vi "Main.vi"(8 "error in (no error)":errorcluster, 11 "ModuleAdmin":refnum<class "ModuleAdmin.lvclass">) -> ()   [LabVIEW 2014, in "AnalysisModule.lvlib"]
uses:
  AnalysisModule.lvlib
  <userlib>/NIST/ModuleAdminLib/ModuleAdmin/ModuleAdmin.lvclass
  AnalysisPlugins/AnalysisPluginBaseClass/Typedefs/clSensorData.ctl
  AnalysisPlugins/AnalysisPluginBaseClass/AnalysisPluginsBase.lvclass/AnalysisPluginsBase.ctl
  PublicAPI/Arguments/Requests/clStopArgument.ctl
  AnalysisPlugins/AnalysisPluginBaseClass/Typedefs/clSampleData.ctl
  AnalysisPlugins/AnalysisPluginBaseClass/Typedefs/clAnalysisConfig.ctl
  AnalysisPlugins/AnalysisPluginBaseClass/Typedefs/SignalParams.ctl
  <userlib>/NIST/ModuleAdminLib/ModuleAdmin/ModuleAdmin.lvclass/ModuleAdmin.ctl
  AnalysisPlugins/AnalysisPluginBaseClass/AnalysisPluginsBase.lvclass
  <userlib>/NIST/BaseClasses/BasePlugin_class/BasePlugin.lvclass/BasePlugin.ctl
  <vilib>/Utility/error.llb/DialogType.ctl
  AnalysisPlugins/AnalysisPluginBaseClass/Accessors/Read ResultArray.vi
  AnalysisPlugins/AnalysisPluginBaseClass/Accessors/Read SampleDataQueName.vi
  AnalysisPlugins/AnalysisPluginBaseClass/Accessors/Write clConfig.vi
  AnalysisPlugins/AnalysisPluginBaseClass/Accessors/Write MagCorr.vi
  AnalysisPlugins/AnalysisPluginBaseClass/Accessors/Write DelayCorr.vi
  AnalysisPlugins/AnalysisPluginBaseClass/Accessors/Write SignalParams.vi
  AnalysisPlugins/AnalysisPluginBaseClass/Accessors/Write TestType.vi
  AnalysisPlugins/AnalysisPluginBaseClass/Accessors/Write FileName.vi
  <userlib>/NIST/ModuleAdminLib/ModuleAdmin/Accessors/Read ShowPanel_.vi
  <userlib>/NIST/ModuleAdminLib/ModuleAdmin/Accessors/Write ShowPanel_.vi
  <userlib>/NIST/BaseClasses/BasePlugin_class/Accessors/Write PluginIniFilePath.vi
  AnalysisPlugins/AnalysisPluginBaseClass/Accessors/Write SampleDataQueName.vi
  <userlib>/NIST/BaseClasses/BasePlugin_class/Accessors/Read PluginIniFilePath.vi
  <userlib>/NIST/ModuleAdminLib/ModuleAdmin/Accessors/Read CloneRegRef.vi
  <vilib>/Utility/error.llb/Error Cluster From Error Code.vi
  <vilib>/ErrorRing/Error Ring.xnode
  <userlib>/NIST/ModuleAdminLib/CloneRegistration/CloneRegistration.lvclass
  <userlib>/NIST/ModuleAdminLib/ModuleAdmin.lvlib
  Sensor/SensorModule/SensorModule.lvlib
panel:
  out "error out":errorcluster
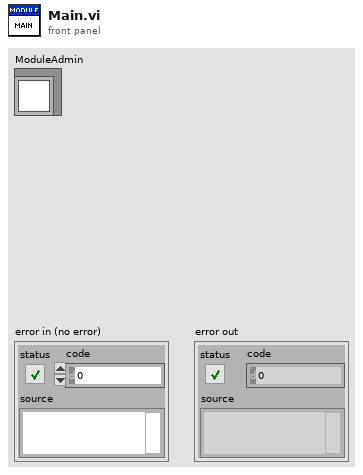
[diagram p1: front panel]
types:
  T1 = typedef "AnalysisPlugins.lvlib/AnalysisPluginsBase.lvclass/clSensorData.ctl" = cluster{"SensorType":string, "SensorData":variant}
  T2 = typedef "AnalysisModule.lvlib/clRequestEvents.ctl" = cluster{"StopRequest":refnum<user-event>, "PathToINI":refnum<user-event>, " LoadPlugin":refnum<user-event>, "ShowPanel":refnum<user-event>, "WriteSamples":refnum<user-event>, "ReadConfig":refnum<user-event>, "WriteConfig":refnum<user-event>, "WriteSignalParams":refnum<user-event>, "WriteTestType":refnum<user-event>, "WriteFileName":refnum<user-event>, "WriteMagCorr":refnum<user-event>, "WriteDlyCorr":refnum<user-event>}
  T3 = typedef "AnalysisModule.lvlib/clBroadcastEvents.ctl" = cluster{"DidInit":refnum<user-event>, "StatusUpdate":refnum<user-event>, "ErrorReport":refnum<user-event>, "DidStop":refnum<user-event>, "PathToINI":refnum<user-event>, "Config":refnum<user-event>, "ResultReport":refnum<user-event>}
  T4 = typedef "SensorModule.lvlib/clBroadcastEvents.ctl" = cluster{"DidInit":refnum<user-event>, "StatusUpdate":refnum<user-event>, "ErrorReport":refnum<user-event>, "DidStop":refnum<user-event>, "PathToINI":refnum<user-event>, "SensorReport":refnum<user-event>, "SensorConfig":refnum<user-event>}
  T5 = typedef "AnalysisModule.lvlib/clStopArgument.ctl" = cluster{"Exit via Stop Module Req?":bool, "Wait for Module to stop?":bool, "ModuleAdmin":refnum<class "ModuleAdmin.lvclass">}
  T6 = typedef "AnalysisPlugins.lvlib/AnalysisPluginsBase.lvclass/clAnalysisConfig.ctl" = cluster{"F0":u32, "SettlingTime":dbl, "AnalysisCycles":dbl, "SampleRate":dbl, "NumChannels":u32, "TsOffset":enum16{"start", "middle", "end"}}
  T7 = typedef "AnalysisPlugins.lvlib/AnalysisPluginsBase.lvclass/SignalParams.ctl" = dbl[]
  T8 = enum32{"Invalid", "Standard", "Closed", "Hidden", "Minimized", "Maximized"}
  T9 = typedef "AnalysisPlugins.lvlib/AnalysisPluginsBase.lvclass/clSampleData.ctl" = cluster{"Timestamp":ext, "SampleDataInput":cluster{"dSampleData":dbl[], "iActualPts":i32}[]}
  T10 = typedef "DialogType.ctl" = u16
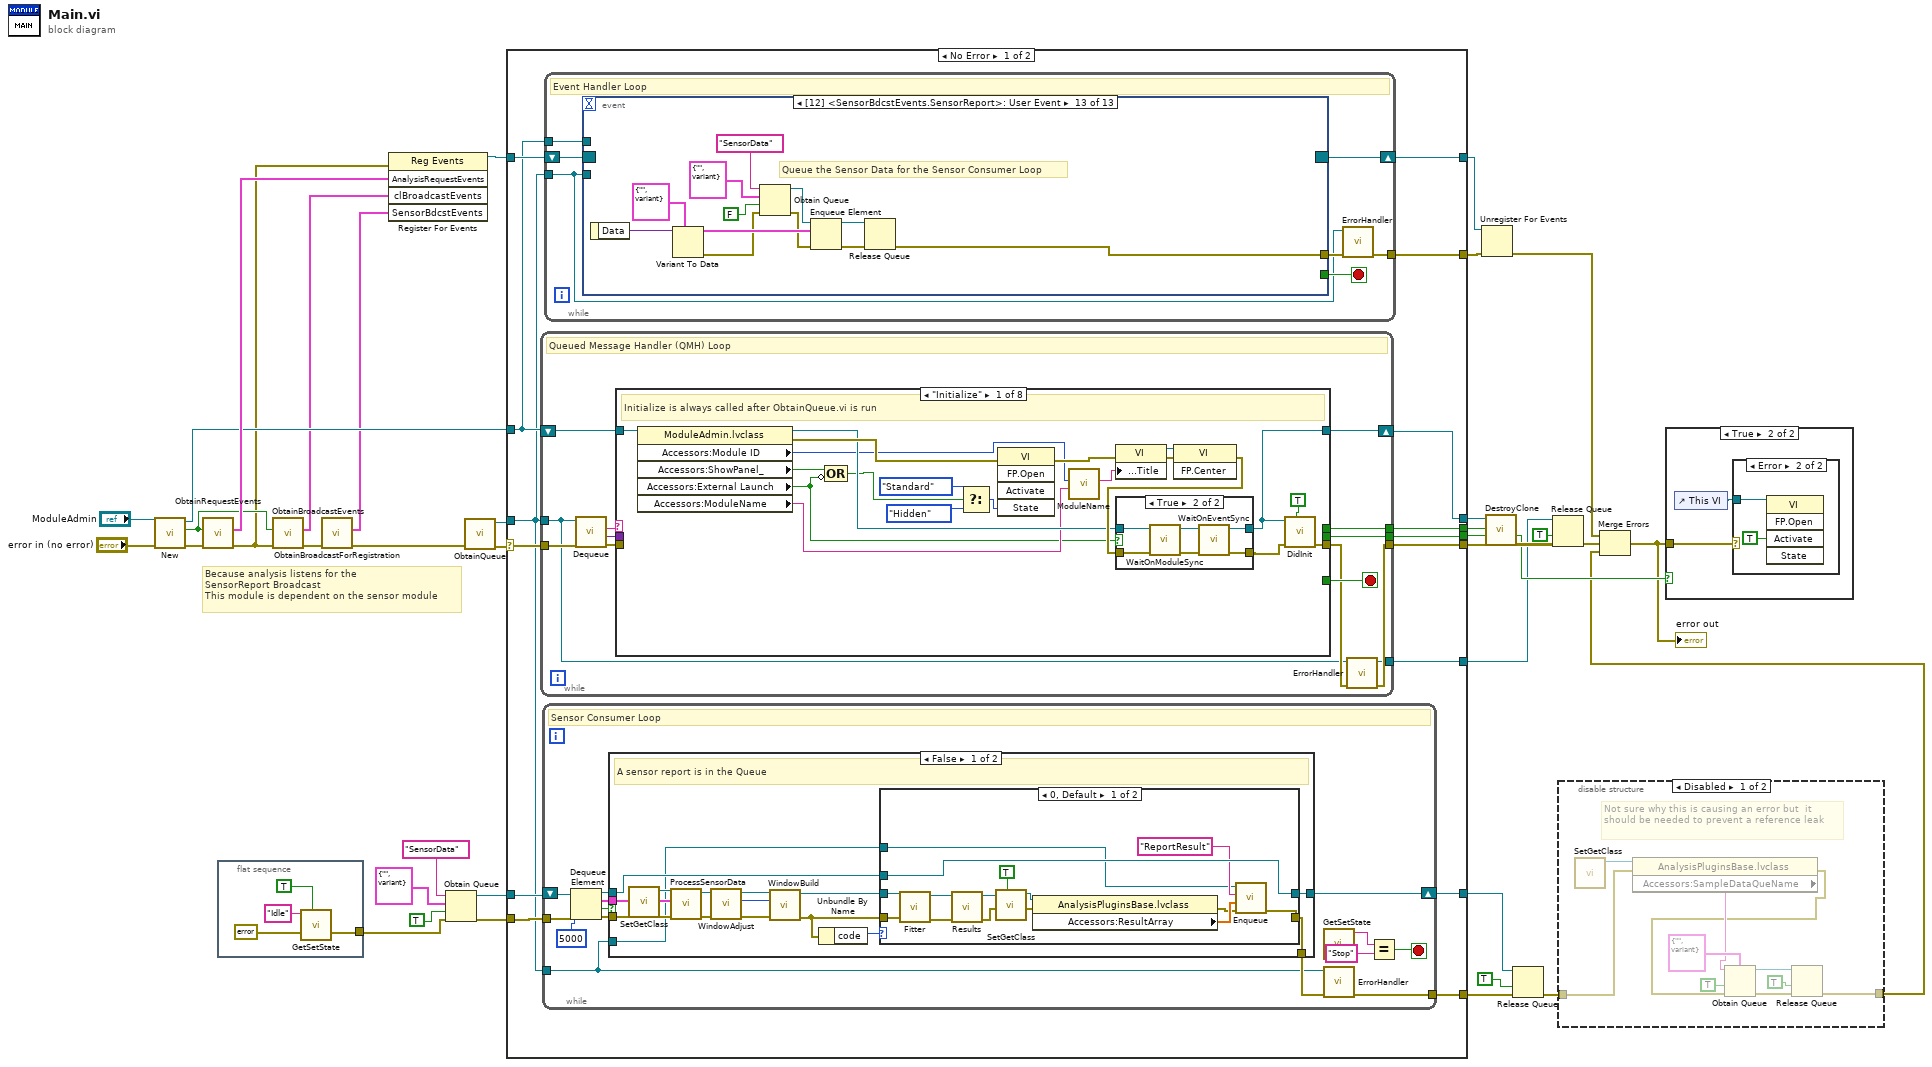
[diagram p0: block diagram]
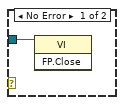
[diagram p4: hidden frame]
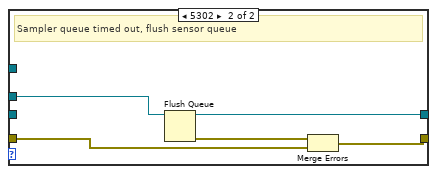
[diagram p5: hidden frame]
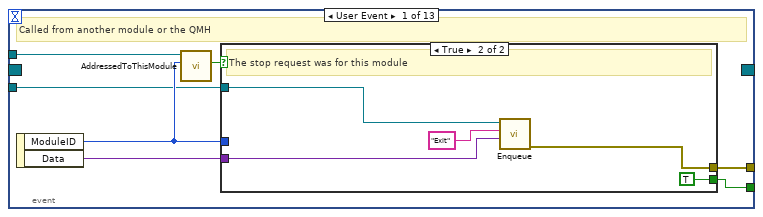
[diagram p7: hidden frame]
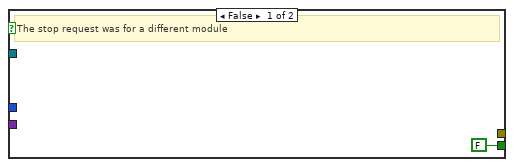
[diagram p8: hidden frame]
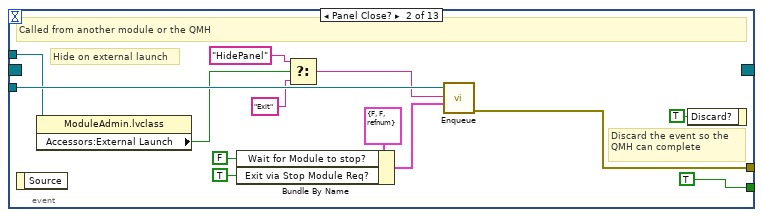
[diagram p9: hidden frame]
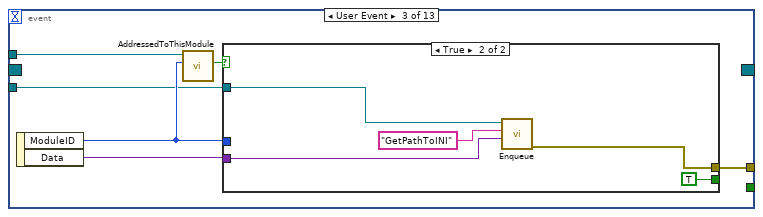
[diagram p10: hidden frame]
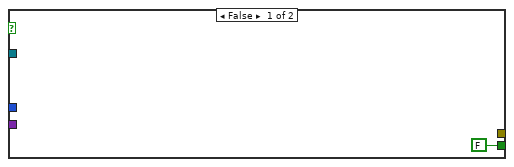
[diagram p11: hidden frame]
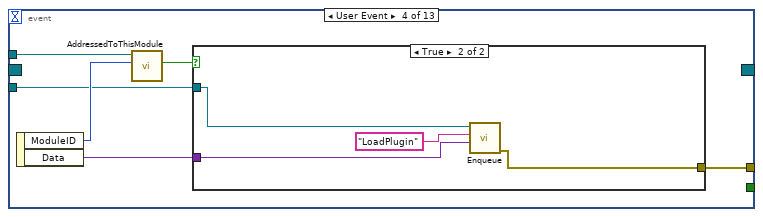
[diagram p12: hidden frame]
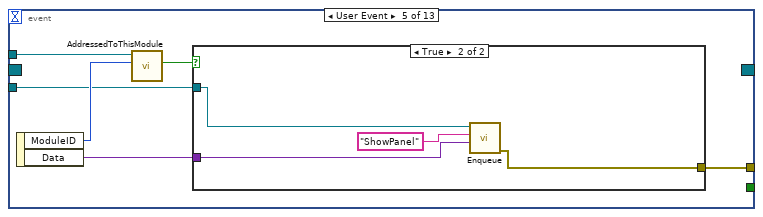
[diagram p14: hidden frame]
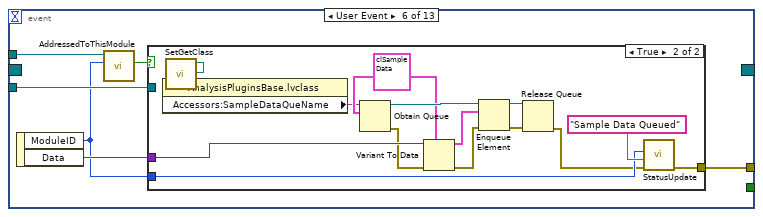
[diagram p16: hidden frame]
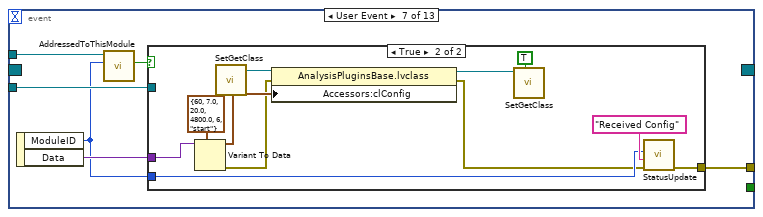
[diagram p18: hidden frame]
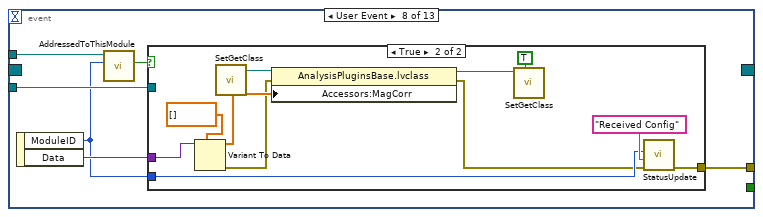
[diagram p20: hidden frame]
diagram:
  # "Because analysis listens for the\nSensorReport Broadcast\nThis module is dependent on the sensor module"
  n1 = call <userlib>:"New.vi"("error in (no error)"="error in (no error)", "ModuleAdmin"="ModuleAdmin") -> ("error out"=w36:errorcluster, "First?"=w31:bool, "ModuleAdmin"=w32:refnum<class "ModuleAdmin.lvclass">)  [unwired: 7 in]
  n2 = call "ObtainRequestEvents.vi"("error in (no error)"=w36, "CreateNew (F)"=w31) -> ("error out"=w30:errorcluster, "AnalysisRequestEvents"=w35:T2)  [unwired: 8 in]
  n3 = flat-sequence {
    tunnel: [errorcluster {"status"=FALSE, "code"=0, "source"=""} ("error constant")] -> w15
    frame #0 {
      n4 = call "GetSetState.vi"("Set (f)"=TRUE, "State In"="Idle") -> ()  [unwired: 9 in, 1 out]
    }
  }
  n5 = call "ObtainBroadcastEvents.vi"("error in (no error)"=w30, "CreateNew? (F)"=w31) -> ("error out"=w14:errorcluster, "clBroadcastEvents"=w29:T3)  [unwired: 8 in]
  n6 = call "ObtainBroadcastForRegistration.vi"("error in (no error)"=w14) -> ("error out"=w13:errorcluster, "SensorBdcstEvents"=w12:T4)  [unwired: 9 in]
  n7 = register-events(error in=w30, w35, w29, w12) -> (reference out=w28:refnum<event-registration>)  [unwired: 1 in, 1 out]
  n8 = Obtain Queue(name (unnamed)="SensorData", element data type=T1 {"SensorType"="", "SensorData"=variant} ("clSensorData"), create if not found? (T)=TRUE, error in (no error)=w15) -> (queue out=w17:refnum<queue>, error out=w16:errorcluster)  [unwired: 1 in, 1 out]
  n9 = call "ObtainQueue.vi"("error in (no error)"=w13) -> ("error out"=w34:errorcluster, "MessageQueue"=w33:refnum<queue>)  [unwired: 9 in]
  n10 = case shown="No Error" w34 {
    selector: w34 -> [w56 w477]
    tunnel: w33 -> [w46 w467]
    tunnel: w32 -> [w53 w474]
    tunnel: [w55 w475] -> w27
    tunnel: w28 -> [w54 w469]
    tunnel: [w52 w473] -> w25
    tunnel: [w51 _] -> w24
    tunnel: [w50 _] -> w23
    tunnel: [w49 _] -> w11
    tunnel: w17 -> [w48 w468]
    tunnel: w16 -> [w47 w470]
    tunnel: [w45 w470] -> w6
    tunnel: [w44 w469] -> w10
    tunnel: [w43 w468] -> w3
    tunnel: [w42 w467] -> w2
    frame No Error {
      n11 = while {
        tunnel: w46 -> [w310]
        tunnel: w56 -> [w319]
        tunnel: [w312] -> w55
        tunnel: [w314] -> w51
        tunnel: [w313] -> w50
        shift-right: [w309] -> w52
        shift-left: w53 -> [w315]
        tunnel: [w308] -> w42
        stop <- w320 stop-if-true
        # "Queued Message Handler (QMH) Loop"
        n12 = call "Dequeue.vi"("error in (no error)"=w319, "MessageQueue"=w310) -> ("error out"=w318:errorcluster, "Message Data"=w316:variant, "Message"=w317:string)  [unwired: 6 in, 1 out]
        n13 = case shown="\"Initialize\"" w317 {
          selector: w317 -> [_ _ _ _ _ _ _ w455]
          tunnel: [_ _ _ _ _ w427 _ _] -> w320
          tunnel: w315 -> [w340 w356 w368 w416 w426 w429 w437 w458]
          tunnel: [w330 w349 w369 w417 w419 w435 w438 w454] -> w311
          tunnel: w318 -> [_ w359 w373 w414 w425 w434 w446 _]
          tunnel: w316 -> [_ w358 w375 _ _ w433 w445 _]
          tunnel: [_ _ _ _ _ w431 _ _] -> w314
          tunnel: [_ _ _ _ _ w430 _ _] -> w313
          tunnel: [w323 w355 w367 w412 w424 w429 w436 w452] -> w309
          frame "Initialize" {
            # "Initialize is always called after ObtainQueue.vi is run"
            n14 = property class="ModuleAdmin.lvclass"(reference=w340) -> (reference out=w328:refnum<class "ModuleAdmin.lvclass">, error out=w337:errorcluster, "Accessors:Module ID"=w322:i32, "Accessors:ShowPanel_"=w326:bool, "Accessors:External Launch"=w325:bool, "Accessors:ModuleName"=w327:string)  [unwired: 1 in]
            n15 = Compound Arithmetic op=OR(w326, invert w325) -> (w324:bool)
            n16 = Select(t=T8."Standard" ("Front Panel Window:State"), s=w324, f=T8."Hidden" ("Front Panel Window:State")) -> (s? t:f=w333:T8)
            n17 = invoke class="VI" method="FP.Open"(error in=w337, "State"=w333) -> (error out=w336:errorcluster)  [unwired: 3 in, 4 out]
            n18 = call <userlib>:"ModuleName.vi"("Name"=w327, "ModuleID"=w322) -> ("ModuleName"=w332:string)  [unwired: 9 in]
            n19 = property class="VI"(error in=w336, "Front Panel.Title"=w332) -> (reference out=w339:refnum<vi>, error out=w338:errorcluster)  [unwired: 1 in]
            n20 = invoke class="VI" method="FP.Center"(reference=w339, error in=w338) -> (error out=w329:errorcluster)  [unwired: 1 in, 2 out]
            n21 = case shown="True" w325 {
              tunnel: [w341 w347] -> w321
              tunnel: [w342 w344] -> w323
              tunnel: w329 -> [w341 w346]
              tunnel: w328 -> [w342 w343]
              frame False {
              }
              frame True {
                n22 = call <userlib>:"WaitOnModuleSync.vi"("error in (no error)"=w346, "ModuleAdmin"=w343) -> ("error out"=w348:errorcluster, "ModuleAdmin"=w345:refnum<class "ModuleAdmin.lvclass">)  [unwired: 8 in]
                n23 = call <userlib>:"WaitOnEventSync.vi"("error in (no error)"=w348, "ModuleAdmin"=w345) -> ("error out"=w347:errorcluster, "ModuleAdmin"=w344:refnum<class "ModuleAdmin.lvclass">)  [unwired: 8 in]
              }
            }
            n24 = call "DidInit.vi"("Init?"=TRUE, "error in (no error)"=w321, "ModuleAdmin"=w323) -> ("error out"=w330:errorcluster)  [unwired: 8 in]
          }
          frame "ShowPanel" {
            n25 = Variant To Data(error in=w359, type=TRUE, Variant=w358) -> (data=w351:bool, error out=w354:errorcluster)
            n26 = Select(t=T8."Standard" ("Front Panel Window:State"), s=w351, f=T8."Hidden" ("Front Panel Window:State")) -> (s? t:f=w350:T8)
            n27 = property class="VI"(error in=w354, "FP.State"=w350) -> (error out=w349:errorcluster)  [unwired: 1 in, 1 out]
            n28 = property class="ModuleAdmin.lvclass"(reference=w356, "Accessors:ShowPanel_"=w351) -> (reference out=w355:refnum<class "ModuleAdmin.lvclass">)  [unwired: 1 in, 1 out]
          }
          frame "LoadPlugin" {
            n29 = Variant To Data(error in=w373, type=path "", Variant=w375) -> (data=w364:path, error out=w363:errorcluster)
            n30 = call "GetDefaultParams.vi"("error in (no error)"=w363, "PathToIni"=w364) -> ("error out"=w362:errorcluster, "clConfig"=w360:T6, "PathToClass"=w361:path)  [unwired: 7 in]
            n31 = call <vilib>:"Check if File or Folder Exists.vi"("error in (no error)"=w362, "path"=w361) -> ("error out"=w370:errorcluster, "file or folder exists?"=w372:bool, "dup path"=w371:path)  [unwired: 7 in]
            n32 = case shown="True" w372 {
              tunnel: w371 -> [w381 w403]
              tunnel: w370 -> [w376 w410]
              tunnel: [w377 w406] -> w369
              tunnel: w368 -> [w380 w405]
              tunnel: [refnum<class "AnalysisPluginsBase.lvclass"> refnum ("AnalysisPlugins.lvlib:AnalysisPluginsBase.lvclass") w391] -> w366
              tunnel: w364 -> [_ w401]
              tunnel: [w380 w400] -> w367
              tunnel: w360 -> [_ w392]
              frame False {
                n33 = Path To String(path=w381) -> (string=w382:string)
                n34 = xnode "Error Ring"("parameter 0"=w382) -> ("error out"=w378:errorcluster)
                n35 = Merge Errors(w376, w378) -> (w377:errorcluster)
              }
              frame True {
                n36 = call-dynamic "LoadClassFromFile.vi"("error in (no error)"=w410, "class path"=w403, "reference in"=refnum<class "AnalysisPluginsBase.lvclass"> refnum) -> ("error out"=w402:errorcluster, "reference out"=w404:refnum<class "AnalysisPluginsBase.lvclass">)  [unwired: 7 in]
                n37 = property class="ModuleAdmin.lvclass"(reference=w405) -> (reference out=w400:refnum<class "ModuleAdmin.lvclass">, "Accessors:Module ID"=w396:i32)  [unwired: 1 in, 1 out]
                n38 = Number To Decimal String(number=w396) -> (decimal integer string=w398:string)  [unwired: 1 in]
                n39 = Concatenate Strings("SampleData" ("name (unnamed)"), w398) -> (w393:string)
                n40 = Obtain Queue(name (unnamed)=w393, element data type=T9 {"Timestamp"=0.0, "SampleDataInput"=[]} ("clSampleData"), create if not found? (T)=TRUE) -> ()  [unwired: 2 in, 3 out]
                n41 = property class="AnalysisPluginsBase.lvclass"(reference=w404, error in=w402, "Accessors:PluginIniFilePath"=w401, "Accessors:SampleDataQueName"=w393, "Accessors:clConfig"=w392) -> (reference out=w391:refnum<class "AnalysisPluginsBase.lvclass">, error out=w390:errorcluster)
                n42 = Path To String(path=w403) -> (string=w408:string)
                n43 = Format Into String(format string="Plugin %s loaded ", w408) -> (resulting string=w407:string)  [unwired: 2 in, 1 out]
                n44 = call "StatusUpdate.vi"("error in (no error)"=w390, "Status"=w407, "ModuleID"=w396) -> ("error out"=w406:errorcluster)  [unwired: 8 in]
              }
            }
            n45 = call "SetGetClass.vi"("Set (f)"=TRUE, "Analysis In"=w366) -> ()  [unwired: 9 in, 1 out]
          }
          frame "GetPathToINI" {
            n46 = call "SetGetClass.vi"() -> ("Analysis Out"=w411:refnum<class "AnalysisPluginsBase.lvclass">)  [unwired: 11 in]
            n47 = property class="AnalysisPluginsBase.lvclass"(reference=w411, error in=w414) -> (error out=w413:errorcluster, "Accessors:PluginIniFilePath"=w415:path)  [unwired: 1 out]
            n48 = property class="ModuleAdmin.lvclass"(reference=w416) -> (reference out=w412:refnum<class "ModuleAdmin.lvclass">, "Accessors:Module ID"=w418:i32)  [unwired: 1 in, 1 out]
            n49 = call "PathToINIBroadcast.vi"("error in (no error)"=w413, "PathToINI"=w415, "ModuleID"=w418) -> ("error out"=w417:errorcluster)  [unwired: 8 in]
          }
          frame "ReportResult" {
            n50 = call "SetGetClass.vi"() -> ("Analysis Out"=w423:refnum<class "AnalysisPluginsBase.lvclass">)  [unwired: 11 in]
            n51 = property class="AnalysisPluginsBase.lvclass"(reference=w423, error in=w425) -> (error out=w420:errorcluster, "Accessors:ResultArray"=w421:dbl[])  [unwired: 1 out]
            n52 = property class="ModuleAdmin.lvclass"(reference=w426) -> (reference out=w424:refnum<class "ModuleAdmin.lvclass">, "Accessors:Module ID"=w422:i32)  [unwired: 1 in, 1 out]
            n53 = call "ReportResults.vi"("error in (no error)"=w420, "ResultsArray"=w421, "ModuleID"=w422) -> ("error out"=w419:errorcluster)  [unwired: 8 in]
          }
          frame "Exit" {
            w427 = TRUE
            # "Called by the StopRequest event handler case"
            n54 = control-ref of="This VI"() -> (w432:refnum<vi>)
            n55 = call "HandleExit.vi"("error in (no error)"=w434, "VI Refnum"=w432, "StopArgument"=w433, "ModuleAdmin"=w429) -> ("error out"=w435:errorcluster, "Exit via Stop Module Req?"=w430:bool, "WaitForStop?"=w431:bool)  [unwired: 5 in]
            n56 = call "GetSetState.vi"("Set (f)"=w427, "State In"="Stop") -> ()  [unwired: 9 in, 1 out]
          }
          frame "Error" {
            n57 = property class="ModuleAdmin.lvclass"(reference=w437) -> (reference out=w436:refnum<class "ModuleAdmin.lvclass">, "Accessors:External Launch"=w441:bool, "Accessors:Module ID"=w439:i32)  [unwired: 1 in, 1 out]
            n58 = Variant To Data(error in=w446, type=errorcluster {"status"=FALSE, "code"=0, "source"=""} ("error constant"), Variant=w445) -> (data=w440:errorcluster, error out=w443:errorcluster)
            n59 = call "ReportError.vi"("error in (no error)"=w443, "ErrorReported"=w440, "ModuleID"=w439) -> ("error out"=w442:errorcluster)  [unwired: 8 in]
            n60 = case shown="False" w441 {
              tunnel: w442 -> [w450 w451]
              tunnel: w440 -> [w449 _]
              tunnel: [w448 w451] -> w438
              tunnel: w437 -> [w447 _]
              frame False {
                # "Todo:  Add an event to ask the user\nIf the module should stop or continue"
                # "Stand alone: now, force an exit"
                n61 = call <vilib>:"Simple Error Handler.vi"("error in (no error)"=w449) -> ()  [unwired: 4 in, 5 out]
                n62 = call "StopRequest.vi"("error in (no error)"=w450, "ModuleAdmin"=w447) -> ("error out"=w448:errorcluster)  [unwired: 8 in, 1 out]
              }
              frame True {
                # "Externally launched modules only broadcast the error msg"
              }
            }
          }
          frame Default {
            # "Called only if a message was queued and no QMH case was created"
            n63 = property class="ModuleAdmin.lvclass"(reference=w458) -> (reference out=w452:refnum<class "ModuleAdmin.lvclass">, "Accessors:Module ID"=w457:i32, "Accessors:ModuleName"=w453:string)  [unwired: 1 in, 1 out]
            n64 = call <userlib>:"ModuleName.vi"("Name"=w453, "ModuleID"=w457) -> ("ModuleName"=w456:string)  [unwired: 9 in]
            n65 = xnode "Error Ring"("parameter 0"=w455, "parameter 1"=w456) -> ("error out"=w454:errorcluster)
          }
        }
        n66 = call "ErrorHandler.vi"("error in (no error)"=w311, "MessageQueue"=w310) -> ("error out"=w312:errorcluster, "MessageQueue"=w308:refnum<queue>)  [unwired: 8 in]
      }
      n67 = while {
        tunnel: w47 -> [w63]
        tunnel: w46 -> [w57]
        tunnel: [w61] -> w45
        shift-right: [w58] -> w43
        shift-left: w48 -> [w60]
        stop <- w68 stop-if-true
        # "Sensor Consumer Loop"
        n68 = Dequeue Element(queue=w60, timeout in ms (-1)=5000, error in (no error)=w63) -> (queue out=w59:refnum<queue>, element=w65:T1, timed out?=w66:bool, error out=w64:errorcluster)
        n69 = case shown="False" w66 {
          tunnel: w65 -> [w77 _]
          tunnel: w64 -> [w85 w106]
          tunnel: [w74 w106] -> w62
          tunnel: w59 -> [w73 w105]
          tunnel: [w72 w105] -> w58
          tunnel: w57 -> [w71 _]
          frame False {
            # "A sensor report is in the Queue"
            n70 = call "SetGetClass.vi"() -> ("Analysis Out"=w84:refnum<class "AnalysisPluginsBase.lvclass">)  [unwired: 11 in]
            n71 = call-dynamic "ProcessSensorData.vi"("error in (no error)"=w85, "clSensorData"=w77, "Class In"=w84) -> ("error out"=w83:errorcluster, "Class Out"=w82:refnum<class "AnalysisPluginsBase.lvclass">)  [unwired: 7 in]
            n72 = call "WindowAdjust.vi"("error in (no error)"=w83, "AnalysisPluginsBase in"=w82) -> ("error out"=w81:errorcluster, "SamplesNeeded"=w79:u32, "AnalysisPluginsBase out"=w80:refnum<class "AnalysisPluginsBase.lvclass">)  [unwired: 7 in]
            n73 = call "WindowBuild.vi"("error in (no error)"=w81, "SamplesNeeded"=w79, "AnalysisPluginsBase in"=w80) -> ("error out"=w75:errorcluster, "AnalysisPluginsBase out"=w76:refnum<class "AnalysisPluginsBase.lvclass">)  [unwired: 7 in]
            n74 = Unbundle By Name(w75) -> ("code"=w78:i32)
            n75 = case shown="0, Default" w78 {
              tunnel: w76 -> [w96 _]
              tunnel: w75 -> [w97 w100]
              tunnel: [w92 w104] -> w74
              tunnel: w73 -> [w98 w103]
              tunnel: [w98 w101] -> w72
              tunnel: w71 -> [w86 _]
              frame 0, Default {
                n76 = call-dynamic "Fitter.vi"("error in (no error)"=w97, "AnalysisPluginsBase in"=w96) -> ("error out"=w95:errorcluster, "AnalysisPluginsBase out"=w94:refnum<class "AnalysisPluginsBase.lvclass">)  [unwired: 8 in]
                n77 = call-dynamic "Results.vi"("error in (no error)"=w95, "AnalysisPluginsBase in"=w94) -> ("error out"=w88:errorcluster, "AnalysisPluginsBase out"=w93:refnum<class "AnalysisPluginsBase.lvclass">)  [unwired: 8 in]
                n78 = call "SetGetClass.vi"("Set (f)"=TRUE, "Analysis In"=w93) -> ("Analysis Out"=w91:refnum<class "AnalysisPluginsBase.lvclass">)  [unwired: 9 in]
                n79 = property class="AnalysisPluginsBase.lvclass"(reference=w91, error in=w88) -> (error out=w87:errorcluster, "Accessors:ResultArray"=w90:dbl[])  [unwired: 1 out]
                n80 = call "Enqueue.vi"("error in (no error)"=w87, "Message Data"=w90, "Message"="ReportResult", "MessageQueue"=w86) -> ("error out"=w92:errorcluster)  [unwired: 6 in, 1 out]
              }
              frame 5302 {
                # "Sampler queue timed out, flush sensor queue"
                n81 = Flush Queue(queue=w103) -> (queue out=w101:refnum<queue>, error out=w102:errorcluster)  [unwired: 1 in, 1 out]
                n82 = Merge Errors(w102, w100) -> (w104:errorcluster)
              }
            }
          }
          frame True {
            # "Queue Timed out, allow the loop to run to check for Stop State"
          }
        }
        n83 = call "GetSetState.vi"() -> ("State Out"=w70:string)  [unwired: 11 in]
        n84 = call "ErrorHandler.vi"("error in (no error)"=w62, "MessageQueue"=w57) -> ("error out"=w61:errorcluster)  [unwired: 8 in, 1 out]
        n85 = Equal?(x=w70, y="Stop") -> (x = y?=w68:bool)
      }
      n86 = while {
        tunnel: w46 -> [w107]
        shift-right: [w111] -> w44
        shift-left: w54 -> [w112]
        tunnel: w53 -> [w110]
        tunnel: [w108] -> w49
        stop <- w113 stop-if-true
        # "Event Handler Loop"
        n87 = event shown="[12] <SensorBdcstEvents.SensorReport>: User Event" {
          selector: w112 -> [_ _ _ _ _ _ _ _ _ _ _ _ _]
          dyn-events: [_ _ _ _ _ _ _ _ _ _ _ _ _] -> w111
          timeout: _ -> [_ _ _ _ _ _ _ _ _ _ _ _ _]
          tunnel: w107 -> [w117 w139 w142 w153 w163 w175 w195 w212 w229 w246 w263 w280 _]
          tunnel: [w116 TRUE _ _ _ _ _ _ _ _ _ _ _] -> w113
          tunnel: w110 -> [w120 w133 w141 w157 w167 w177 w197 w214 w231 w248 w265 w282 _]
          tunnel: [w115 w137 w140 w154 w164 w173 w193 w210 w227 w244 w261 w278 w297] -> w109
          event User Event {
            # "Called from another module or the QMH"
            n88 = event-data() -> ("ModuleID"=w118:i32, "Data"=w114:variant)  [unwired: 1 in]
            n89 = call <userlib>:"AddressedToThisModule.vi"("ModuleID"=w118, "ModuleAdmin"=w120) -> ("AddressedToThisInstance?"=w119:bool)  [unwired: 8 in, 1 out]
            n90 = case shown="True" w119 {
              tunnel: w118 -> [_ _]
              tunnel: w117 -> [_ w126]
              tunnel: [FALSE TRUE] -> w116
              tunnel: [_ w124] -> w115
              tunnel: w114 -> [_ w122]
              frame False {
                # "The stop request was for a different module"
              }
              frame True {
                # "The stop request was for this module"
                n91 = call "Enqueue.vi"("Message Data"=w122, "Message"="Exit", "MessageQueue"=w126) -> ("error out"=w124:errorcluster)  [unwired: 7 in, 1 out]
              }
            }
          }
          event Panel Close? {
            # "Hide on external launch"
            # "Discard the event so the QMH can complete"
            # "Called from another module or the QMH"
            n92 = event-data() -> ()  [unwired: 1 in, 1 out]
            n93 = property class="ModuleAdmin.lvclass"(reference=w133) -> ("Accessors:External Launch"=w128:bool)  [unwired: 1 in, 2 out]
            n94 = Bundle By Name(cluster=T5 {"Exit via Stop Module Req?"=FALSE, "Wait for Module to stop?"=FALSE, "ModuleAdmin"=refnum} ("Stop Argument"), "Wait for Module to stop?"=FALSE, "Exit via Stop Module Req?"=TRUE) -> (w134:T5)
            n95 = Select(t="HidePanel", s=w128, f="Exit" ("Message")) -> (s? t:f=w130:string)
            n96 = call "Enqueue.vi"("Message Data"=w134, "Message"=w130, "MessageQueue"=w139) -> ("error out"=w137:errorcluster)  [unwired: 7 in, 1 out]
            n97 = event-data("Discard?"=TRUE) -> ()  [unwired: 1 in, 1 out]
          }
          event User Event {
            n98 = event-data() -> ("ModuleID"=w143:i32, "Data"=w144:variant)  [unwired: 1 in]
            n99 = call <userlib>:"AddressedToThisModule.vi"("ModuleID"=w143, "ModuleAdmin"=w141) -> ("AddressedToThisInstance?"=w145:bool)  [unwired: 8 in, 1 out]
            n100 = case shown="True" w145 {
              tunnel: w143 -> [_ _]
              tunnel: w142 -> [_ w151]
              tunnel: [FALSE TRUE] -> _
              tunnel: [_ w149] -> w140
              tunnel: w144 -> [_ w147]
              frame False {
                # "The stop request was for a different module"
              }
              frame True {
                # "The stop request was for this module"
                n101 = call "Enqueue.vi"("Message Data"=w147, "Message"="GetPathToINI", "MessageQueue"=w151) -> ("error out"=w149:errorcluster)  [unwired: 7 in, 1 out]
              }
            }
          }
          event User Event {
            n102 = event-data() -> ("ModuleID"=w156:i32, "Data"=w152:variant)  [unwired: 1 in]
            n103 = call <userlib>:"AddressedToThisModule.vi"("ModuleID"=w156, "ModuleAdmin"=w157) -> ("AddressedToThisInstance?"=w155:bool)  [unwired: 8 in, 1 out]
            n104 = case shown="True" w155 {
              tunnel: [_ w158] -> w154
              tunnel: w153 -> [_ w161]
              tunnel: w152 -> [_ w159]
              frame False {
              }
              frame True {
                n105 = call "Enqueue.vi"("Message Data"=w159, "Message"="LoadPlugin", "MessageQueue"=w161) -> ("error out"=w158:errorcluster)  [unwired: 7 in, 1 out]
              }
            }
          }
          event User Event {
            n106 = event-data() -> ("ModuleID"=w166:i32, "Data"=w162:variant)  [unwired: 1 in]
            n107 = call <userlib>:"AddressedToThisModule.vi"("ModuleID"=w166, "ModuleAdmin"=w167) -> ("AddressedToThisInstance?"=w165:bool)  [unwired: 8 in, 1 out]
            n108 = case shown="True" w165 {
              tunnel: [_ w168] -> w164
              tunnel: w163 -> [_ w171]
              tunnel: w162 -> [_ w169]
              frame False {
              }
              frame True {
                n109 = call "Enqueue.vi"("Message Data"=w169, "Message"="ShowPanel", "MessageQueue"=w171) -> ("error out"=w168:errorcluster)  [unwired: 7 in, 1 out]
              }
            }
          }
          event User Event {
            n110 = event-data() -> ("ModuleID"=w172:i32, "Data"=w174:variant)  [unwired: 1 in]
            n111 = call <userlib>:"AddressedToThisModule.vi"("ModuleID"=w172, "ModuleAdmin"=w177) -> ("AddressedToThisInstance?"=w176:bool)  [unwired: 8 in, 1 out]
            n112 = case shown="True" w176 {
              tunnel: w175 -> [_ _]
              tunnel: w174 -> [_ w191]
              tunnel: [_ w184] -> w173
              tunnel: w172 -> [_ w183]
              frame False {
              }
              frame True {
                w188 = T9 {"Timestamp"=0.0, "SampleDataInput"=[]} ("clSampleData")
                n113 = call "SetGetClass.vi"() -> ("Analysis Out"=w182:refnum<class "AnalysisPluginsBase.lvclass">)  [unwired: 11 in]
                n114 = property class="AnalysisPluginsBase.lvclass"(reference=w182) -> ("Accessors:SampleDataQueName"=w181:string)  [unwired: 1 in, 2 out]
                n115 = Obtain Queue(name (unnamed)=w181, element data type=w188) -> (queue out=w189:refnum<queue>, error out=w187:errorcluster)  [unwired: 3 in, 1 out]
                n116 = Variant To Data(error in=w187, type=w188, Variant=w191) -> (data=w190:T9, error out=w186:errorcluster)
                n117 = Enqueue Element(queue=w189, element=w190, error in (no error)=w186) -> (queue out=w178:refnum<queue>, error out=w180:errorcluster)  [unwired: 1 in, 1 out]
                n118 = Release Queue(queue=w178, error in (no error)=w180) -> (error out=w179:errorcluster)  [unwired: 1 in, 2 out]
                n119 = call "StatusUpdate.vi"("error in (no error)"=w179, "Status"="Sample Data Queued", "ModuleID"=w183) -> ("error out"=w184:errorcluster)  [unwired: 8 in]
              }
            }
          }
          event User Event {
            n120 = event-data() -> ("ModuleID"=w192:i32, "Data"=w194:variant)  [unwired: 1 in]
            n121 = call <userlib>:"AddressedToThisModule.vi"("ModuleID"=w192, "ModuleAdmin"=w197) -> ("AddressedToThisInstance?"=w196:bool)  [unwired: 8 in, 1 out]
            n122 = case shown="True" w196 {
              tunnel: w195 -> [_ _]
              tunnel: w194 -> [_ w208]
              tunnel: [_ w206] -> w193
              tunnel: w192 -> [_ w205]
              frame False {
              }
              frame True {
                n123 = Variant To Data(type=T6 {"F0"=60, "SettlingTime"=7.0, "AnalysisCycles"=20.0, "SampleRate"=4800.0, "NumChannels"=6, "TsOffset"=enum."start"} ("clAnalysisConfig"), Variant=w208) -> (data=w202:T6, error out=w199:errorcluster)  [unwired: 1 in]
                n124 = call "SetGetClass.vi"() -> ("Analysis Out"=w203:refnum<class "AnalysisPluginsBase.lvclass">)  [unwired: 11 in]
                n125 = property class="AnalysisPluginsBase.lvclass"(reference=w203, error in=w199, "Accessors:clConfig"=w202) -> (reference out=w200:refnum<class "AnalysisPluginsBase.lvclass">, error out=w198:errorcluster)
                n126 = call "SetGetClass.vi"("Set (f)"=TRUE, "Analysis In"=w200) -> ()  [unwired: 9 in, 1 out]
                n127 = call "StatusUpdate.vi"("error in (no error)"=w198, "Status"="Received Config", "ModuleID"=w205) -> ("error out"=w206:errorcluster)  [unwired: 8 in]
              }
            }
          }
          event User Event {
            n128 = event-data() -> ("ModuleID"=w209:i32, "Data"=w211:variant)  [unwired: 1 in]
            n129 = call <userlib>:"AddressedToThisModule.vi"("ModuleID"=w209, "ModuleAdmin"=w214) -> ("AddressedToThisInstance?"=w213:bool)  [unwired: 8 in, 1 out]
            n130 = case shown="True" w213 {
              tunnel: w212 -> [_ _]
              tunnel: w211 -> [_ w225]
              tunnel: [_ w223] -> w210
              tunnel: w209 -> [_ w222]
              frame False {
              }
              frame True {
                n131 = Variant To Data(type=dbl[] [], Variant=w225) -> (data=w220:dbl[], error out=w217:errorcluster)  [unwired: 1 in]
                n132 = call "SetGetClass.vi"() -> ("Analysis Out"=w221:refnum<class "AnalysisPluginsBase.lvclass">)  [unwired: 11 in]
                n133 = property class="AnalysisPluginsBase.lvclass"(reference=w221, error in=w217, "Accessors:MagCorr"=w220) -> (reference out=w218:refnum<class "AnalysisPluginsBase.lvclass">, error out=w216:errorcluster)
                n134 = call "SetGetClass.vi"("Set (f)"=TRUE, "Analysis In"=w218) -> ()  [unwired: 9 in, 1 out]
                n135 = call "StatusUpdate.vi"("error in (no error)"=w216, "Status"="Received Config", "ModuleID"=w222) -> ("error out"=w223:errorcluster)  [unwired: 8 in]
              }
            }
          }
          event User Event {
            n136 = event-data() -> ("ModuleID"=w226:i32, "Data"=w228:variant)  [unwired: 1 in]
            n137 = call <userlib>:"AddressedToThisModule.vi"("ModuleID"=w226, "ModuleAdmin"=w231) -> ("AddressedToThisInstance?"=w230:bool)  [unwired: 8 in, 1 out]
            n138 = case shown="True" w230 {
              tunnel: w229 -> [_ _]
              tunnel: w228 -> [_ w242]
              tunnel: [_ w240] -> w227
              tunnel: w226 -> [_ w239]
              frame False {
              }
              frame True {
                n139 = Variant To Data(type=dbl[] [], Variant=w242) -> (data=w237:dbl[], error out=w234:errorcluster)  [unwired: 1 in]
                n140 = call "SetGetClass.vi"() -> ("Analysis Out"=w238:refnum<class "AnalysisPluginsBase.lvclass">)  [unwired: 11 in]
                n141 = property class="AnalysisPluginsBase.lvclass"(reference=w238, error in=w234, "Accessors:DelayCorr"=w237) -> (reference out=w235:refnum<class "AnalysisPluginsBase.lvclass">, error out=w233:errorcluster)
                n142 = call "SetGetClass.vi"("Set (f)"=TRUE, "Analysis In"=w235) -> ()  [unwired: 9 in, 1 out]
                n143 = call "StatusUpdate.vi"("error in (no error)"=w233, "Status"="Received Config", "ModuleID"=w239) -> ("error out"=w240:errorcluster)  [unwired: 8 in]
              }
            }
          }
          event User Event {
            n144 = event-data() -> ("ModuleID"=w243:i32, "Data"=w245:variant)  [unwired: 1 in]
            n145 = call <userlib>:"AddressedToThisModule.vi"("ModuleID"=w243, "ModuleAdmin"=w248) -> ("AddressedToThisInstance?"=w247:bool)  [unwired: 8 in, 1 out]
            n146 = case shown="True" w247 {
              tunnel: w246 -> [_ _]
              tunnel: w245 -> [_ w259]
              tunnel: [_ w257] -> w244
              tunnel: w243 -> [_ w256]
              frame False {
              }
              frame True {
                n147 = Variant To Data(type=T7 [] ("SignalParams"), Variant=w259) -> (data=w254:T7, error out=w251:errorcluster)  [unwired: 1 in]
                n148 = call "SetGetClass.vi"() -> ("Analysis Out"=w255:refnum<class "AnalysisPluginsBase.lvclass">)  [unwired: 11 in]
                n149 = property class="AnalysisPluginsBase.lvclass"(reference=w255, error in=w251, "Accessors:SignalParams"=w254) -> (reference out=w252:refnum<class "AnalysisPluginsBase.lvclass">, error out=w250:errorcluster)
                n150 = call "SetGetClass.vi"("Set (f)"=TRUE, "Analysis In"=w252) -> ()  [unwired: 9 in, 1 out]
                n151 = call "StatusUpdate.vi"("error in (no error)"=w250, "Status"="Received Signal Params", "ModuleID"=w256) -> ("error out"=w257:errorcluster)  [unwired: 8 in]
              }
            }
          }
          event User Event {
            n152 = event-data() -> ("ModuleID"=w260:i32, "Data"=w262:variant)  [unwired: 1 in]
            n153 = call <userlib>:"AddressedToThisModule.vi"("ModuleID"=w260, "ModuleAdmin"=w265) -> ("AddressedToThisInstance?"=w264:bool)  [unwired: 8 in, 1 out]
            n154 = case shown="True" w264 {
              tunnel: w263 -> [_ _]
              tunnel: w262 -> [_ w276]
              tunnel: [_ w274] -> w261
              tunnel: w260 -> [_ w273]
              frame False {
              }
              frame True {
                n155 = Variant To Data(type="", Variant=w276) -> (data=w271:string, error out=w268:errorcluster)  [unwired: 1 in]
                n156 = call "SetGetClass.vi"() -> ("Analysis Out"=w272:refnum<class "AnalysisPluginsBase.lvclass">)  [unwired: 11 in]
                n157 = property class="AnalysisPluginsBase.lvclass"(reference=w272, error in=w268, "Accessors:TestType"=w271) -> (reference out=w269:refnum<class "AnalysisPluginsBase.lvclass">, error out=w267:errorcluster)
                n158 = call "SetGetClass.vi"("Set (f)"=TRUE, "Analysis In"=w269) -> ()  [unwired: 9 in, 1 out]
                n159 = call "StatusUpdate.vi"("error in (no error)"=w267, "Status"="Received TestType", "ModuleID"=w273) -> ("error out"=w274:errorcluster)  [unwired: 8 in]
              }
            }
          }
          event User Event {
            n160 = event-data() -> ("ModuleID"=w277:i32, "Data"=w279:variant)  [unwired: 1 in]
            n161 = call <userlib>:"AddressedToThisModule.vi"("ModuleID"=w277, "ModuleAdmin"=w282) -> ("AddressedToThisInstance?"=w281:bool)  [unwired: 8 in, 1 out]
            n162 = case shown="True" w281 {
              tunnel: w280 -> [_ _]
              tunnel: w279 -> [_ w295]
              tunnel: [_ w293] -> w278
              tunnel: w277 -> [_ w292]
              frame False {
              }
              frame True {
                n163 = Variant To Data(type="", Variant=w295) -> (data=w290:string, error out=w288:errorcluster)  [unwired: 1 in]
                n164 = call "SetGetClass.vi"() -> ("Analysis Out"=w291:refnum<class "AnalysisPluginsBase.lvclass">)  [unwired: 11 in]
                n165 = property class="AnalysisPluginsBase.lvclass"(reference=w291, error in=w288, "Accessors:FileName"=w290) -> (reference out=w286:refnum<class "AnalysisPluginsBase.lvclass">, error out=w284:errorcluster)
                n166 = call-dynamic "InitResultFile.vi"("error in (no error)"=w284, "AnalysisPluginsBase in"=w286) -> ("error out"=w283:errorcluster, "AnalysisPluginsBase out"=w285:refnum<class "AnalysisPluginsBase.lvclass">)  [unwired: 8 in]
                n167 = call "SetGetClass.vi"("Set (f)"=TRUE, "Analysis In"=w285) -> ()  [unwired: 9 in, 1 out]
                n168 = call "StatusUpdate.vi"("error in (no error)"=w283, "Status"="Results File Initialized", "ModuleID"=w292) -> ("error out"=w293:errorcluster)  [unwired: 8 in]
              }
            }
          }
          event User Event {
            # "Queue the Sensor Data for the Sensor Consumer Loop"
            n169 = event-data() -> ("Data"=w307:variant)  [unwired: 1 in]
            n170 = Variant To Data(type=T1 {"SensorType"="", "SensorData"=variant} ("clSensorData"), Variant=w307) -> (data=w301:T1, error out=w300:errorcluster)  [unwired: 1 in]
            n171 = Obtain Queue(name (unnamed)="SensorData", element data type=T1 {"SensorType"="", "SensorData"=variant} ("clSensorData"), create if not found? (T)=FALSE, error in (no error)=w300) -> (queue out=w302:refnum<queue>, error out=w299:errorcluster)  [unwired: 1 in, 1 out]
            n172 = Enqueue Element(queue=w302, element=w301, error in (no error)=w299) -> (queue out=w296:refnum<queue>, error out=w298:errorcluster)  [unwired: 1 in, 1 out]
            n173 = Release Queue(queue=w296, error in (no error)=w298) -> (error out=w297:errorcluster)  [unwired: 1 in, 2 out]
          }
        }
        n174 = call "ErrorHandler.vi"("error in (no error)"=w109, "MessageQueue"=w107) -> ("error out"=w108:errorcluster)  [unwired: 8 in, 1 out]
      }
    }
    frame Error {
      n175 = property class="ModuleAdmin.lvclass"(reference=w474) -> (reference out=w473:refnum<class "ModuleAdmin.lvclass">, "Accessors:CloneRegRef"=w472:refnum<data-value>, "Accessors:Module ID"=w471:i32)  [unwired: 1 in, 1 out]
      n176 = call <userlib>:"Remove.vi"("Module ID"=w471, "CloneRegRef"=w472) -> ("error out"=w476:errorcluster)  [unwired: 7 in, 2 out]
      n177 = flat-sequence {
        tunnel: w477 -> [w480]
        tunnel: w476 -> [_]
        tunnel: [w478] -> w475
        frame #0 {
          w479 = T10 2 items=["no dialog", "OK message", "continue or stop message", "OK message + warnings", "continue/stop + warnings"] ("type of dialog (OK msg:1)")
          n178 = call <vilib>:"Simple Error Handler.vi"("type of dialog (OK msg:1)"=w479, "error in (no error)"=w480) -> ("error out"=w478:errorcluster)  [unwired: 3 in, 4 out]
        }
      }
    }
  }
  n179 = Unregister For Events(event registration refnum=w10, error in=w11) -> (error out=w8:errorcluster)
  n180 = call "DestroyClone.vi"("error in (no error)"=w27, "Exit via Stop Module Req?"=w23, "Wait for Module to stop?"=w24, "ModuleAdmin"=w25) -> ("error out"=w26:errorcluster, "External Launch"=w22:bool)  [unwired: 5 in, 1 out]
  n181 = Release Queue(queue=w3, force destroy? (F)=TRUE, error in (no error)=w6) -> (error out=w1:errorcluster)  [unwired: 2 out]
  n182 = Release Queue(queue=w2, force destroy? (F)=TRUE, error in (no error)=w26) -> (error out=w21:errorcluster)  [unwired: 2 out]
  n183 = disable-structure shown="Disabled" {
    disable-tunnel: [w487 _] -> w7
    disable-tunnel: w1 -> [w482 _]
    frame Disabled {
      # "Not sure why this is causing an error but  it should be needed to prevent a reference leak"
      n184 = call "SetGetClass.vi"() -> ("Analysis Out"=w485:refnum<class "AnalysisPluginsBase.lvclass">)  [unwired: 11 in]
      n185 = property class="AnalysisPluginsBase.lvclass"(reference=w485, error in=w482) -> (error out=w481:errorcluster, "Accessors:SampleDataQueName"=w484:string)  [unwired: 1 out]
      n186 = Obtain Queue(name (unnamed)=w484, element data type=T1 {"SensorType"="", "SensorData"=variant} ("clSensorData"), create if not found? (T)=TRUE, error in (no error)=w481) -> (queue out=w490:refnum<queue>, error out=w489:errorcluster)  [unwired: 1 in, 1 out]
      n187 = Release Queue(queue=w490, force destroy? (F)=TRUE, error in (no error)=w489) -> (error out=w487:errorcluster)  [unwired: 2 out]
    }
    frame Enabled {
    }
  }
  n188 = Merge Errors(w8, w21, w7) -> (w9:errorcluster)
  "error out" <- w9
  n189 = case shown="True" w22 {
    tunnel: w9 -> [_ w492]
    frame False {
    }
    frame True {
      n190 = control-ref of="This VI"() -> (w491:refnum<vi>)
      n191 = case shown="Error" w492 {
        tunnel: w491 -> [w493 w494]
        frame No Error {
          n192 = invoke class="VI" method="FP.Close"(reference=w493) -> ()  [unwired: 2 in, 3 out]
        }
        frame Error {
          n193 = invoke class="VI" method="FP.Open"(reference=w494, "Activate"=TRUE ("Activate?")) -> ()  [unwired: 3 in, 5 out]
        }
      }
    }
  }
